vi "簇处理.vi"() -> ()   [LabVIEW 2018]
panel:
  out "大小":i32
  in  "确定按钮":bool
  out "detail":string[](array[string])
  out "lenght":dbl[](array[numeric])
  out "start":dbl[](array[numeric])
  out "abort":bool[](array[boolean])
  out "title":string[](array[string])
  out "act":bool[](array[boolean])
  in  "修改通道选择":enum16{"1", "2", "3", "4", "5", "6"}(ring)
  in  "修改":T1
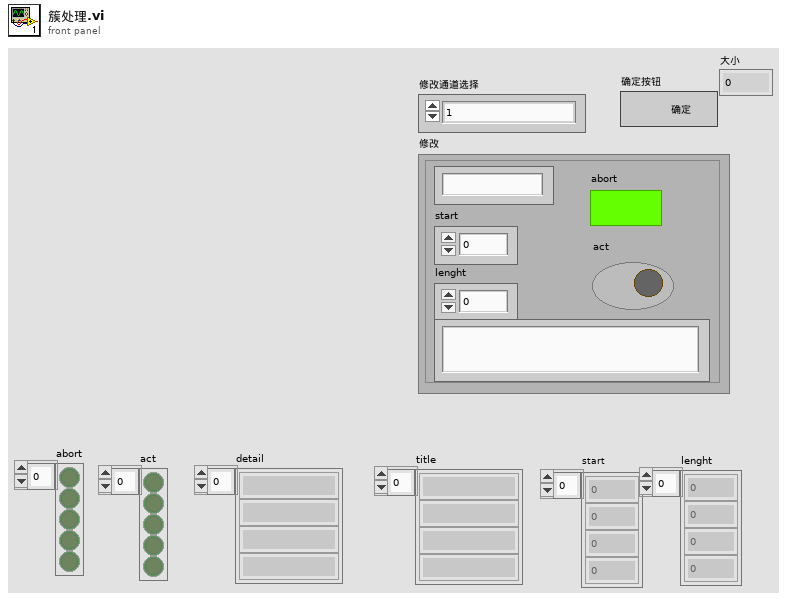
[diagram p1: front panel]
types:
  T1 = cluster{"title":string, "abort":bool, "act":bool, "start":dbl, "lenght":dbl, "detail":string}
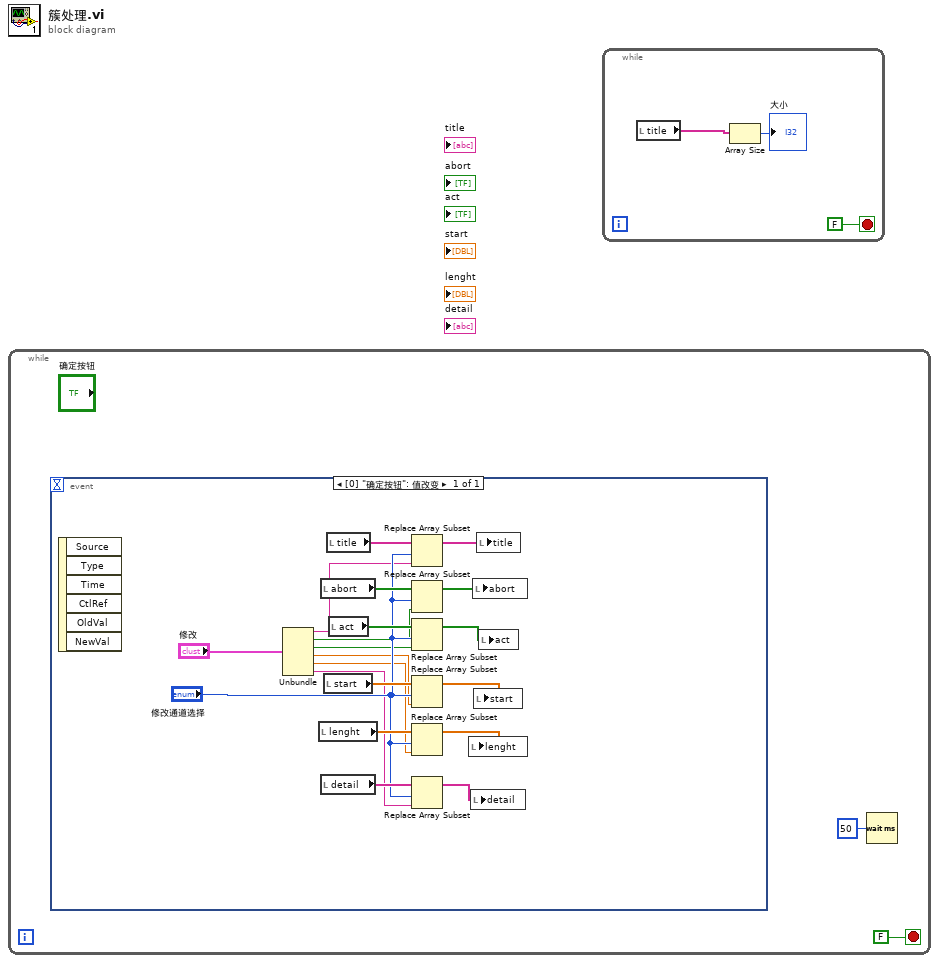
[diagram p0: block diagram]
diagram:
  n1 = while {
    stop <- FALSE stop-if-true
    n2 = event shown="[0] \"确定按钮\": 值改变" {
      selector: _ -> [_]
      dyn-events: _ -> [_]
      timeout: _ -> [_]
      event "确定按钮": Value Change {
        n3 = event-data() -> ()  [unwired: 1 in, 6 out]
        n4 = Unbundle("修改") -> ("title"=w15:string, "abort"=w7:bool, "act"=w6:bool, "start"=w5:dbl, "lenght"=w4:dbl, "detail"=w3:string)
        n5 = local read "lenght"() -> (w18:dbl[])
        n6 = local read "abort"() -> (w21:bool[])
        n7 = local read "detail"() -> (w17:string[])
        n8 = local read "start"() -> (w19:dbl[])
        n9 = local read "title"() -> (w22:string[])
        n10 = local read "act"() -> (w20:bool[])
        n11 = Replace Array Subset(array=w22, new element=w15, index="修改通道选择") -> (w14:string[])
        n12 = Replace Array Subset(array=w21, new element=w7, index="修改通道选择") -> (w13:bool[])
        n13 = Replace Array Subset(array=w20, new element=w6, index="修改通道选择") -> (w12:bool[])
        n14 = Replace Array Subset(array=w19, new element=w5, index="修改通道选择") -> (w11:dbl[])
        n15 = Replace Array Subset(array=w18, new element=w4, index="修改通道选择") -> (w10:dbl[])
        n16 = Replace Array Subset(array=w17, new element=w3, index="修改通道选择") -> (w9:string[])
        n17 = local write "lenght"(w10) -> ()
        n18 = local write "detail"(w9) -> ()
        n19 = local write "abort"(w13) -> ()
        n20 = local write "start"(w11) -> ()
        n21 = local write "title"(w14) -> ()
        n22 = local write "act"(w12) -> ()
      }
    }
    n23 = Wait (ms)(milliseconds to wait=u32 50 ("等待时间（毫秒）")) -> ()  [unwired: 1 out]
  }
  n24 = while {
    stop <- FALSE stop-if-true
    n25 = local read "title"() -> (w25:string[])
    n26 = Array Size(array=w25) -> (size(s)=→"大小":i32)
  }
